vi "Lift To Inch.vi"(7 "Speed":dbl=0.95, 11 "Inches to move":dbl) -> (2 "Done":bool=TRUE)   [LabVIEW 2014]
uses:
  Begin/Global Variables.vi
  <vilib>/Rock Robotics/Network Tables/SD Write Boolean.vi
  Begin/Global RefNums.vi
  <vilib>/Rock Robotics/Network Tables/SD Write Number.vi
panel:
  in  "Down Speed":dbl=0.75
  in  "homing right PID":T1={"proportional gain (Kc)"=0.0007, "integral time (Ti, min)"=0.0, "derivative time (Td, min)"=0.0003} {"derivative time (Td, min)" format="%.4f"; "integral time (Ti, min)" format="%.6f"; "proportional gain (Kc)" format="%.5f"}
  in  "homing left PID":T2={"proportional gain (Kc)"=0.002, "integral time (Ti, min)"=0.0, "derivative time (Td, min)"=0.0005} {"derivative time (Td, min)" format="%.10f"; "proportional gain (Kc)" format="%.5f"}
  in  "Output Range 2":cluster{"output high":dbl, "output low":dbl}={"output high"=0.5, "output low"=-0.5} {"output low" format="%.2f"; "output high" format="%.2f"}
  in  "Increase":dbl=0.3 format="%#_13g"
  in  "lower limit 2":dbl=0.5 format="%#_13g"
  in  "lower limit":dbl=0.5
  in  "normalize":dbl=0.834
  in  "inches slowed":dbl=10.0
  in  "Dec Constant":dbl=-2.0
  in  "slave offset":dbl=1800.0
  in  "Ramp right PID gains":T1={"proportional gain (Kc)"=0.0006, "integral time (Ti, min)"=0.0, "derivative time (Td, min)"=0.0} {"derivative time (Td, min)" format="%.4f"; "integral time (Ti, min)" format="%.6f"; "proportional gain (Kc)" format="%.5f"}
  in  "Ramp left PID gains":T2={"proportional gain (Kc)"=0.0046, "integral time (Ti, min)"=0.005499999970197678, "derivative time (Td, min)"=0.0001} {"derivative time (Td, min)" format="%.10f"; "proportional gain (Kc)" format="%.5f"}
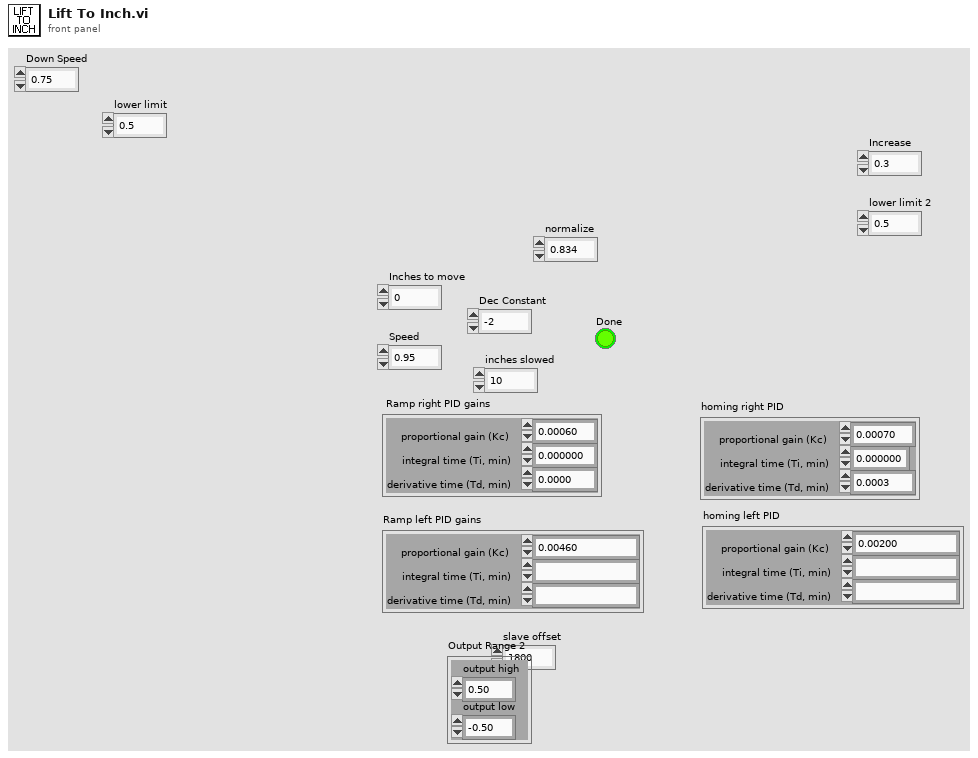
[diagram p1: front panel]
types:
  T1 = cluster{"proportional gain (Kc)":dbl, "integral time (Ti, min)":dbl, "derivative time (Td, min)":dbl}
  T2 = cluster{"proportional gain (Kc)":dbl, "integral time (Ti, min)":fxp<+/-,64,32>, "derivative time (Td, min)":dbl}
  T3 = typedef "WPI_EncoderDevRef.ctl" = cluster{"DevStatus":errorcluster, "EncoderIndex":T4, "CounterIndex":T5, "DistancePerCount":dbl, "Decoding Type":T6}
  T4 = typedef "FPGA_EncoderIdx.ctl" = enum8{"Enc 0", "Enc 1", "Enc 2", "Enc 3", "Enc 4", "Enc 5", "Enc 6", "Enc 7", "Invalid"}
  T5 = typedef "FPGA_CounterCtrSystemIndex.ctl" = enum8{"Ctr 0", "Ctr 1", "Ctr 2", "Ctr 3", "Ctr 4", "Ctr 5", "Ctr 6", "Ctr 7", "Invalid"}
  T6 = typedef "WPI_EncoderType.ctl" = enum16{"1x", "2x", "4x"}
  T7 = typedef "WPI_MotorControlDeviceRef.ctl" = cluster{"DeviceStatus":errorcluster, "Type":T8, "PWM":cluster{"Controller":T9, "PWM Channel":T10, "DeadBand":T11}, "CAN":cluster{"Device Number":u8, "Control Mode":T12, "Semaphore":T13, "Max Vout":dbl, "TalonSRX Control Mode":T14}, "Invert":bool, "TransformRef":T15, "InvTransformRef":T15}
  T8 = typedef "WPI_MotorControlType.ctl" = enum16{"PWM", "CAN", "CANTalonSRX"}
  T9 = typedef "FPGA_TypedefDigitalModule.ctl" = enum16{"Controller 1"}
  T10 = typedef "FPGA_DIOPWMChannel.ctl" = enum8{"PWM 0", "PWM 1", "PWM 2", "PWM 3", "PWM 4", "PWM 5", "PWM 6", "PWM 7", "PWM 8", "PWM 9", "PWM MXP 0", "PWM MXP 1", "PWM MXP 2", "PWM MXP 3", "PWM MXP 4", "PWM MXP 5", "PWM MXP 6", "PWM MXP 7", "PWM MXP 8", "PWM MXP 9", "Invalid"}
  T11 = typedef "WPI_PWMDeadband.ctl" = cluster{"Name":string, "maxPositivePwm":i32, "minPositivePwm":i32, "centerPwm":i32, "maxNegativePwm":i32, "minNegativePwm":i32, "angularRange":u16}
  T12 = typedef "WPI_CANJaguar_ControlMode.ctl" = enum8{"Percent VBus", "Current", "Speed", "Position", "Voltage"}
  T13 = typedef "Semaphore RefNum" = refnum<k1>
  T14 = typedef "WPI_CANTalonSRX_APIControlMode.ctl" = enum8{"Percent VBus", "Speed", "Position", "Slave", "Unchanged / Invalid"}
  T15 = typedef "WPI_PWMTransform_ConPane.ctl" = refnum<vi>
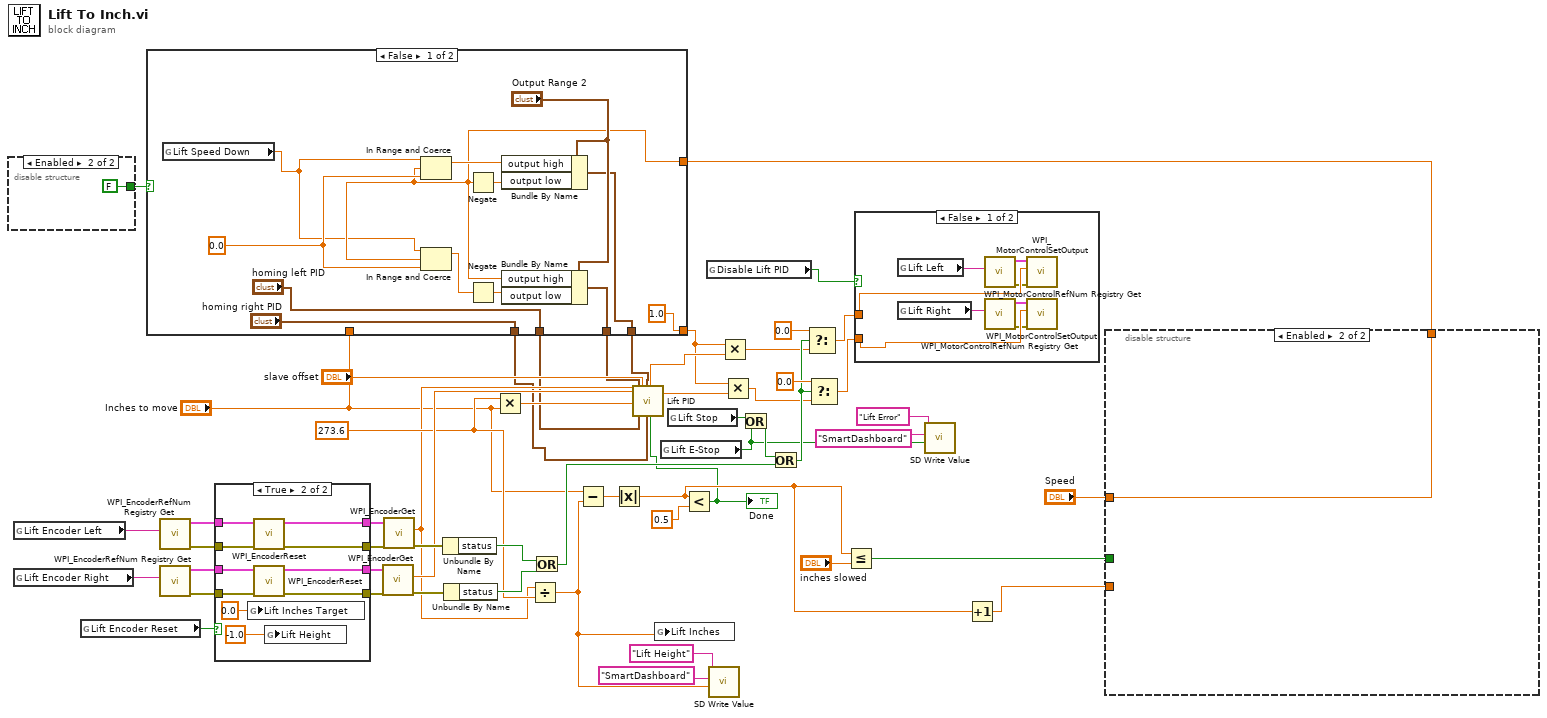
[diagram p0: block diagram]
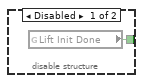
[diagram p2: hidden frame]
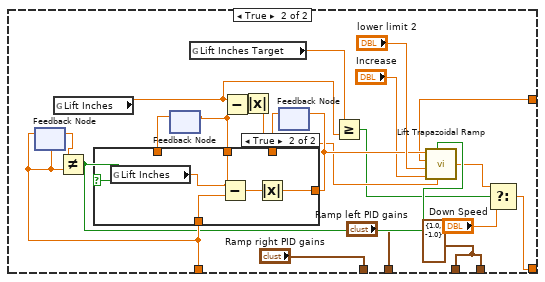
[diagram p3: hidden frame]
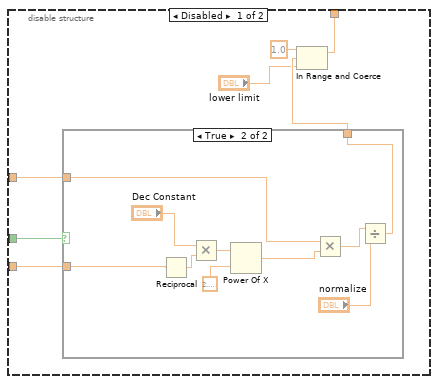
[diagram p6: hidden frame]
diagram:
  w23 = 273.6 ("y")
  n1 = disable-structure shown="Enabled" {
    disable-tunnel: [w56 FALSE ("Lift Init Done")] -> w7
    frame Disabled {
      n2 = global read "Global Variables.vi" "Lift Init Done"() -> (w56:bool)
    }
    frame Enabled {
    }
  }
  n3 = global read "Global RefNums.vi" "Lift Encoder Left"() -> (w33:string)
  n4 = global read "Global RefNums.vi" "Lift Encoder Right"() -> (w32:string)
  n5 = global read "Global Variables.vi" "Lift Encoder Reset"() -> (w22:bool)
  n6 = call <vilib>:"WPI_EncoderRefNum Registry Get.vi"("refnum name"=w33) -> ("error out"=w50:errorcluster, "EncoderDevRef"=w49:T3)  [unwired: 9 in]
  n7 = call <vilib>:"WPI_EncoderRefNum Registry Get.vi"("refnum name"=w32) -> ("error out"=w47:errorcluster, "EncoderDevRef"=w48:T3)  [unwired: 9 in]
  n8 = case shown="True" w22 {
    tunnel: w47 -> [w58 w71]
    tunnel: w48 -> [w59 w70]
    tunnel: w50 -> [w60 w68]
    tunnel: w49 -> [w61 w69]
    tunnel: [w61 w67] -> w52
    tunnel: [w59 w66] -> w53
    tunnel: [w58 w65] -> w54
    tunnel: [w60 w64] -> w55
    frame False {
    }
    frame True {
      n9 = global write "Global Variables.vi" "Lift Inches Target"(0.0 ("Lift Inches Target")) -> ()
      n10 = call <vilib>:"WPI_EncoderReset.vi"("error in (no error)"=w68, "EncoderDevRef"=w69) -> ("error out"=w64:errorcluster, "EncoderDevRef"=w67:T3)  [unwired: 8 in]
      n11 = call <vilib>:"WPI_EncoderReset.vi"("error in (no error)"=w71, "EncoderDevRef"=w70) -> ("error out"=w65:errorcluster, "EncoderDevRef"=w66:T3)  [unwired: 8 in]
      n12 = global write "Global Variables.vi" "Lift Height"(-1.0 ("Lift Inches Target")) -> ()
    }
  }
  n13 = call <vilib>:"WPI_EncoderGet.vi"("error in (no error)"=w54, "EncoderDevRef"=w53) -> ("error out"=w37:errorcluster, "Distance"=w30:dbl)  [unwired: 4 in, 4 out]
  n14 = call <vilib>:"WPI_EncoderGet.vi"("error in (no error)"=w55, "EncoderDevRef"=w52) -> ("error out"=w40:errorcluster, "Distance"=w21:dbl)  [unwired: 4 in, 4 out]
  n15 = Unbundle By Name(w40) -> ("status"=w38:bool)
  n16 = Unbundle By Name(w37) -> ("status"=w36:bool)
  n17 = Multiply(x=w23, y="Inches to move") -> (x*y=w46:dbl)
  n18 = Divide(x=w21, y=w23) -> (x/y=w27:dbl)
  n19 = Or(x=w38, y=w36) -> (x .or. y?=w35:bool)
  n20 = Subtract(x="Inches to move", y=w27) -> (x-y=w45:dbl)
  n21 = Absolute Value(x=w45) -> (abs(x)=w18:dbl)
  n22 = global write "Global Variables.vi" "Lift Inches"(w27) -> ()
  n23 = global read "Global Variables.vi" "Lift E-Stop"() -> (w24:bool)
  n24 = global read "Global Variables.vi" "Lift Stop"() -> (w31:bool)
  n25 = Less?(x=w18, y=0.5) -> (x < y?=w2:bool)
  "Done" <- w2
  n26 = global read "Global Variables.vi" "Disable Lift PID"() -> (w14:bool)
  n27 = call-poly <vilib>:"SD Write Value.vi"("Numeric"=w27, "Table Prefix"="SmartDashboard", "Name"="Lift Height") -> ()  [unwired: 7 in, 2 out]
  n28 = Or(x=w31, y=w24) -> (x .or. y?=w34:bool)
  n29 = Or(x=w34, y=w35) -> (x .or. y?=w39:bool)
  n30 = Less Or Equal?(x=w18, y="inches slowed") -> (x <= y?=w20:bool)
  n31 = call-poly <vilib>:"SD Write Value.vi"("Boolean"=w24, "Table Prefix"="SmartDashboard", "Name"="Lift Error") -> ()  [unwired: 7 in, 2 out]
  n32 = Increment(x=w18) -> (x+1=w17:dbl)
  n33 = disable-structure shown="Enabled" {
    disable-tunnel: w20 -> [w78 _]
    disable-tunnel: "Speed" -> [w77 w90]
    disable-tunnel: w17 -> [w76 _]
    disable-tunnel: [w72 w90] -> w15
    frame Disabled {
      n34 = case shown="True" w78 {
        tunnel: w77 -> [w79 w86]
        tunnel: [w79 w81] -> w75
        tunnel: w76 -> [_ w84]
        frame False {
        }
        frame True {
          n35 = Reciprocal(x=w84) -> (1/x=w83:dbl)
          n36 = Multiply(x="Dec Constant", y=w83) -> (x*y=w87:dbl)
          n37 = Power Of X(1:2.718281828459045, 2:w87) -> (0:w85:dbl)
          n38 = Multiply(x=w86, y=w85) -> (x*y=w82:dbl)
          n39 = Divide(x=w82, y="normalize") -> (x/y=w81:dbl)
        }
      }
      n40 = In Range and Coerce(upper limit=1.0, x=w75, lower limit="lower limit") -> (coerced(x)=w72:dbl)  [unwired: 1 out]
    }
    frame Enabled {
    }
  }
  n41 = case shown="False" w7 {
    tunnel: w15 -> [w95 w108]
    tunnel: [w97 w113] -> w5
    tunnel: "Inches to move" -> [_ w124]
    tunnel: [1.0 ("Speed") w104] -> w10
    tunnel: [w94 w113] -> w6
    tunnel: ["homing left PID" "Ramp left PID gains"] -> w4
    tunnel: ["homing right PID" "Ramp right PID gains"] -> w3
    frame False {
      w101 = 0.0 ("lower limit")
      n42 = global read "Global Variables.vi" "Lift Speed Down"() -> (w91:dbl)
      n43 = In Range and Coerce(upper limit=w91, x=w95, lower limit=w101) -> (coerced(x)=w98:dbl)  [unwired: 1 out]
      n44 = In Range and Coerce(upper limit=w91, x=w95, lower limit=w101) -> (coerced(x)=w102:dbl)  [unwired: 1 out]
      n45 = Negate(x=w95) -> (-x=w99:dbl)
      n46 = Negate(x=w102) -> (-x=w103:dbl)
      n47 = Bundle By Name(cluster="Output Range 2", "output high"=w98, "output low"=w99) -> (w97:cluster{"output high":dbl, "output low":dbl})
      n48 = Bundle By Name(cluster="Output Range 2", "output high"=w95, "output low"=w103) -> (w94:cluster{"output high":dbl, "output low":dbl})
    }
    frame True {
      w113 = cluster{"output high":dbl, "output low":dbl} {"output high"=1.0, "output low"=-1.0} ("left output range")
      n49 = feedback #1(w124) -> (w120:dbl)
      n50 = feedback-in #1(w124) -> ()
      n51 = global read "Global Variables.vi" "Lift Inches"() -> (w110:dbl)
      n52 = Not Equal?(x=w120, y=w124) -> (x != y?=w114:bool)
      n53 = feedback #2() -> (w118:dbl)  [unwired: 1 in]
      n54 = global read "Global Variables.vi" "Lift Inches Target"() -> (w109:dbl)
      n55 = feedback #3() -> (w121:dbl)  [unwired: 1 in]
      n56 = case shown="True" w114 {
        tunnel: w124 -> [_ w129]
        tunnel: [w126 w128] -> w122
        tunnel: w121 -> [w126 _]
        tunnel: [w125 w127] -> w119
        tunnel: w118 -> [w125 _]
        frame False {
        }
        frame True {
          n57 = global read "Global Variables.vi" "Lift Inches"() -> (w127:dbl)
          n58 = Subtract(x=w127, y=w129) -> (x-y=w130:dbl)
          n59 = Absolute Value(x=w130) -> (abs(x)=w128:dbl)
        }
      }
      n60 = feedback-in #2(w119) -> ()
      n61 = Subtract(x=w110, y=w119) -> (x-y=w117:dbl)
      n62 = Absolute Value(x=w117) -> (abs(x)=w116:dbl)
      n63 = feedback-in #3(w122) -> ()
      n64 = Greater Or Equal?(x=w109, y=w110) -> (x >= y?=w106:bool)
      n65 = call "Lift Trapazoidal Ramp.vi"("Encoder"=w116, "Reset"=w114, "Increase"="Increase", "lower limit"="lower limit 2", "Speed (-1 to 1)"=w108, "Distance (inches)"=w122) -> ("Speed"=w107:dbl)
      n66 = Select(t=w107, s=w106, f="Down Speed") -> (s? t:f=w104:dbl)
    }
  }
  n67 = call "Lift PID.vi"("left encoder"=w21, "right encoder"=w30, "move to distance"=w46, "left output range"=w6, "left PID gains"=w4, "slave offset"="slave offset", "right output range"=w5, "right PID gains"=w3, "Reinitialize"=w2) -> ("lift motor left"=w12:dbl, "lift motor right"=w11:dbl)  [unwired: 17 in]
  n68 = Multiply(x=w10, y=w12) -> (x*y=w9:dbl)
  n69 = Multiply(x=w10, y=w11) -> (x*y=w8:dbl)
  n70 = Select(t=0.0, s=w39, f=w9) -> (s? t:f=w42:dbl)
  n71 = Select(t=0.0, s=w39, f=w8) -> (s? t:f=w41:dbl)
  n72 = case shown="False" w14 {
    tunnel: w42 -> [w138 _]
    tunnel: w41 -> [w137 _]
    frame False {
      n73 = global read "Global RefNums.vi" "Lift Left"() -> (w132:string)
      n74 = global read "Global RefNums.vi" "Lift Right"() -> (w131:string)
      n75 = call <vilib>:"WPI_MotorControlRefNum Registry Get.vi"("refnum name"=w132) -> ("error out"=w136:errorcluster, "MotorControlDevRef"=w135:T7)  [unwired: 9 in]
      n76 = call <vilib>:"WPI_MotorControlRefNum Registry Get.vi"("refnum name"=w131) -> ("error out"=w133:errorcluster, "MotorControlDevRef"=w134:T7)  [unwired: 9 in]
      n77 = call <vilib>:"WPI_MotorControlSetOutput.vi"("error in (no error)"=w136, "Output"=w138, "MotorControlDevRef"=w135) -> ()  [unwired: 6 in, 3 out]
      n78 = call <vilib>:"WPI_MotorControlSetOutput.vi"("error in (no error)"=w133, "Output"=w137, "MotorControlDevRef"=w134) -> ()  [unwired: 6 in, 3 out]
    }
    frame True {
    }
  }
